vi "UploadProjects.vi"(8 "error in (no error)":errorcluster, 11 "DB in":refnum<class "DB.lvclass">) -> (0 "error out":errorcluster, 3 "DB out":refnum<class "DB.lvclass">)   [LabVIEW 2015, in "DB.lvclass"]
uses:
  DB.lvclass
  DB.lvclass/DB.ctl
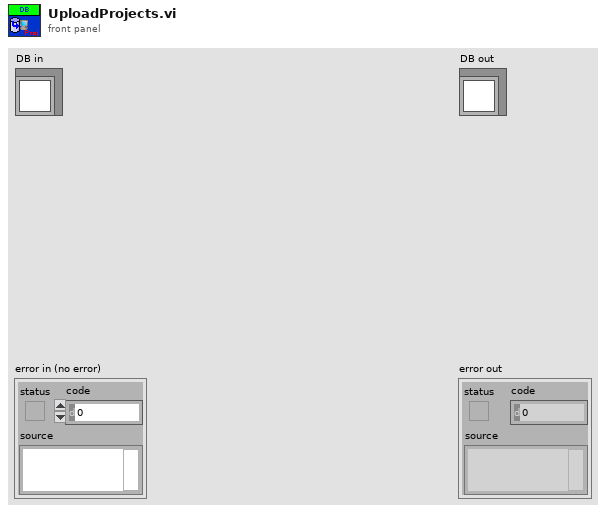
[diagram p1: front panel]
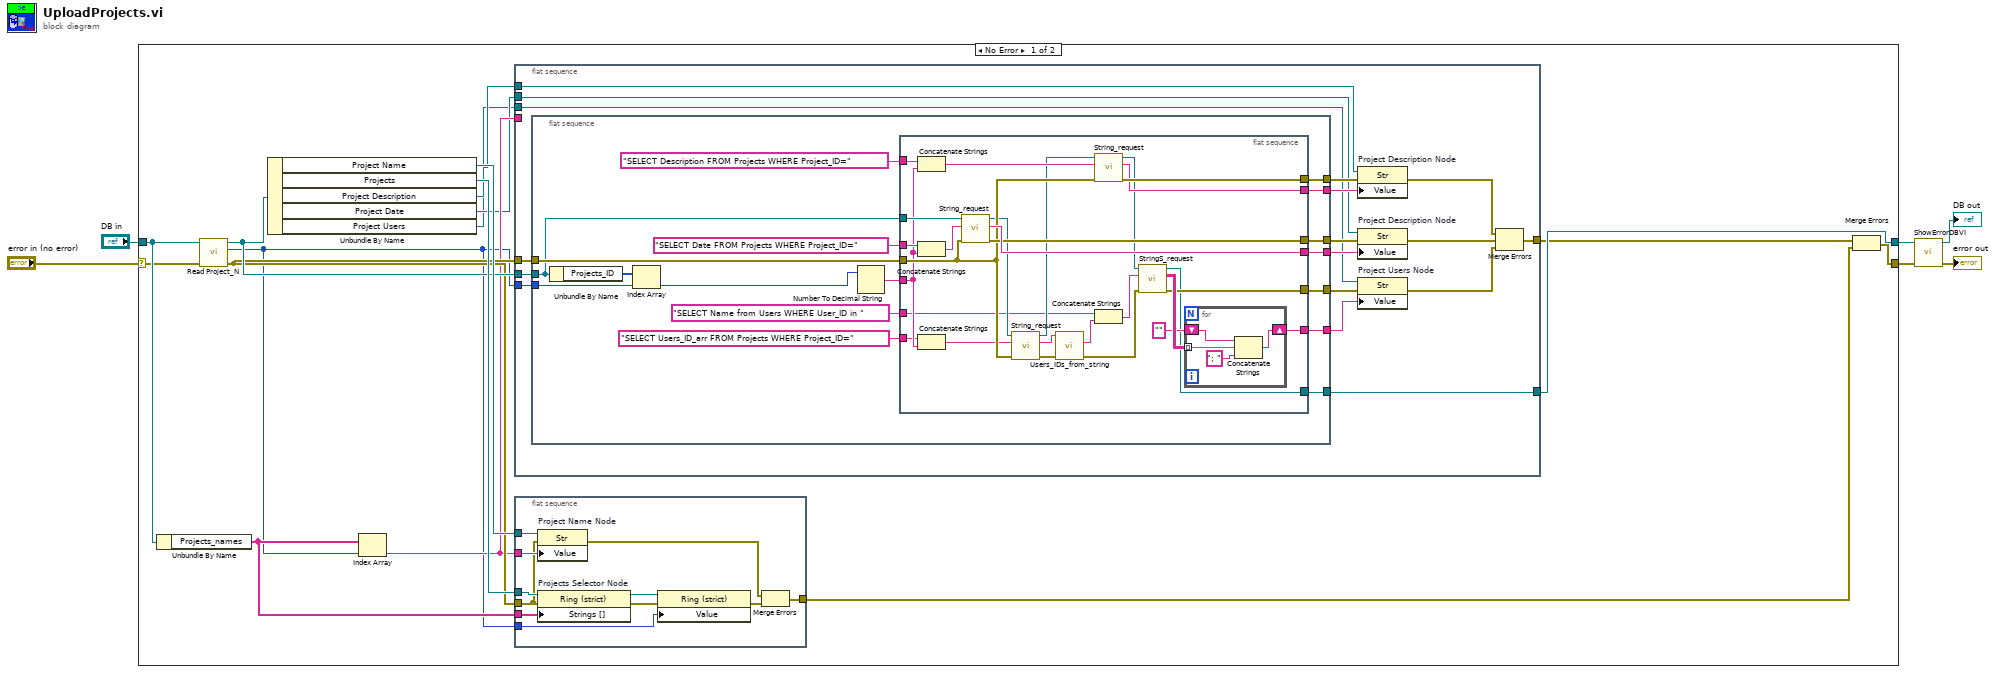
[diagram p0: block diagram]
diagram:
  n1 = case shown="No Error" "error in (no error)" {
    selector: "error in (no error)" -> [w21 w100]
    tunnel: [w11 w100] -> w4
    tunnel: [w10 w99] -> w3
    tunnel: "DB in" -> [w22 w99]
    frame No Error {
      n2 = Unbundle By Name(w22) -> ("Projects_names"=w19:string[])
      n3 = call "Read Project_N.vi"("error in (no error)"=w21, "DB in"=w22) -> ("error out"=w16:errorcluster, "Project_N"=w12:i16, "DB out"=w17:refnum<class "DB.lvclass">)  [unwired: 7 in]
      n4 = Unbundle By Name(w17) -> ("Project Name"=w20:refnum<vi>, "Projects"=w18:refnum<vi>, "Project Description"=w15:refnum<vi>, "Project Date"=w13:refnum<vi>, "Project Users"=w9:refnum<vi>)
      n5 = Index Array(array=w19, index=w12) -> (element=w14:string)
      n6 = flat-sequence {
        tunnel: w17 -> [w40]
        tunnel: [w50] -> w10
        tunnel: w16 -> [w42]
        tunnel: w15 -> [w48]
        tunnel: [w44] -> w8
        tunnel: w14 -> [_]
        tunnel: w13 -> [w46]
        tunnel: w12 -> [w39]
        tunnel: w9 -> [w35]
        frame #0 {
          n7 = flat-sequence {
            tunnel: [w67] -> w50
            tunnel: [w65] -> w49
            tunnel: [w64] -> w47
            tunnel: w42 -> [w63]
            tunnel: [w61] -> w41
            tunnel: w40 -> [w60]
            tunnel: w39 -> [w58]
            tunnel: [w55] -> w38
            tunnel: [w54] -> w36
            tunnel: [w52] -> w34
            frame #0 {
              n8 = Unbundle By Name(w60) -> ("Projects_ID"=w59:i16[])
              n9 = Index Array(array=w59, index=w58) -> (element=w57:i16)
              n10 = Number To Decimal String(number=w57) -> (decimal integer string=w56:string)  [unwired: 1 in]
              n11 = flat-sequence {
                tunnel: [w69] -> w67
                tunnel: "SELECT Description FROM Projects WHERE Project_ID=" ("SQL request") -> [w94]
                tunnel: [w92] -> w65
                tunnel: [w91] -> w64
                tunnel: w63 -> [w85]
                tunnel: "SELECT Date FROM Projects WHERE Project_ID=" ("SQL request") -> [w90]
                tunnel: [w88] -> w61
                tunnel: w60 -> [w86]
                tunnel: w56 -> [w84]
                tunnel: [w87] -> w55
                tunnel: [w73] -> w54
                tunnel: "SELECT Users_ID_arr FROM Projects WHERE Project_ID=" ("SQL request") -> [w83]
                tunnel: [w74] -> w52
                tunnel: "SELECT Name from Users WHERE User_ID in " -> [w68]
                frame #0 {
                  n12 = Concatenate Strings(w94, w84) -> (w93:string)
                  n13 = Concatenate Strings(w90, w84) -> (w89:string)
                  n14 = Concatenate Strings(w83, w84) -> (w82:string)
                  n15 = call-dynamic "String_request.vi"("error in (no error)"=w85, "SQL request"=w89, "DB in"=w86) -> ("error out"=w87:errorcluster, "Result"=w88:string, "DB out"=w72:refnum<class "DB.lvclass">)  [unwired: 6 in]
                  n16 = call-dynamic "String_request.vi"("error in (no error)"=w85, "SQL request"=w82, "DB in"=w72) -> ("error out"=w81:errorcluster, "Result"=w79:string, "DB out"=w71:refnum<class "DB.lvclass">)  [unwired: 6 in]
                  n17 = call "Users_IDs_from_string.vi"("error in"=w81, "input string"=w79) -> ("error out"=w80:errorcluster, "Preformed string"=w78:string)  [unwired: 7 in, 1 out]
                  n18 = call-dynamic "String_request.vi"("error in (no error)"=w85, "SQL request"=w93, "DB in"=w71) -> ("error out"=w92:errorcluster, "Result"=w91:string, "DB out"=w70:refnum<class "DB.lvclass">)  [unwired: 6 in]
                  n19 = Concatenate Strings(w68, w78) -> (w77:string)
                  n20 = call-dynamic "StringS_request.vi"("error in (no error)"=w80, "SQL request"=w77, "DB in"=w70) -> ("error out"=w73:errorcluster, "Result Set"=w76:string[][], "DB out"=w69:refnum<class "DB.lvclass">)  [unwired: 5 in, 1 out]
                  n21 = for {
                    tunnel: w76 -> [w97] mode=indexing
                    shift-right: [w95] -> w74
                    shift-left: "" ("Preformed string") -> [w98]
                    n22 = Concatenate Strings(w98, w97, "; " ("string")) -> (w95:string)
                  }
                }
              }
            }
          }
          n23 = property on="Project Description Node" class="Str"(reference=w48, error in=w49, "Value"=w47) -> (error out=w45:errorcluster)  [unwired: 1 out]
          n24 = property on="Project Description Node" class="Str"(reference=w46, error in=w38, "Value"=w41) -> (error out=w43:errorcluster)  [unwired: 1 out]
          n25 = property on="Project Users Node" class="Str"(reference=w35, error in=w36, "Value"=w34) -> (error out=w37:errorcluster)  [unwired: 1 out]
          n26 = Merge Errors(w45, w43, w37) -> (w44:errorcluster)
        }
      }
      n27 = flat-sequence {
        tunnel: w20 -> [w32]
        tunnel: w19 -> [w31]
        tunnel: w14 -> [w30]
        tunnel: w18 -> [w29]
        tunnel: w12 -> [w27]
        tunnel: w16 -> [w26]
        tunnel: [w23] -> w7
        frame #0 {
          n28 = property on="Project Name Node" class="Str"(reference=w32, error in=w26, "Value"=w30) -> (error out=w25:errorcluster)  [unwired: 1 out]
          n29 = property on="Projects Selector Node" class="Ring (strict)"(reference=w29, error in=w26, "Strings []"=w31) -> (reference out=w33:refnum<vi>, error out=w28:errorcluster)
          n30 = property class="Ring (strict)"(reference=w33, error in=w28, "Value"=w27) -> (error out=w24:errorcluster)  [unwired: 1 out]
          n31 = Merge Errors(w25, w24) -> (w23:errorcluster)
        }
      }
      n32 = Merge Errors(w8, w7) -> (w11:errorcluster)
    }
    frame Error {
    }
  }
  n33 = call "ShowErrorDBVI.vi"("error in (no error)"=w4, "DB in"=w3) -> ("error out"=→"error out":errorcluster, "DB out"=→"DB out":refnum<class "DB.lvclass">)  [unwired: 8 in]
